vi "Feedback Node - Building an Array.vi"() -> ()   [LabVIEW 2023]
doc: "This VI uses a While Loop with a Feedback Node to build an array of random data. A Waveform Graph displays the array of random data as the array is built."
panel:
  out "Random Data (Shift Register)":dbl[](graph)
  out "Random Data (Feedback Node)":dbl[](graph)
  in  "Stop":bool
  # "Overview: Demonstrates the use of a Feedback Node to store data between iterations of a loop.\nInstructions:\nRun the VI. It will display data accumulated across all iterations of a loop. See the block diagram for more information."
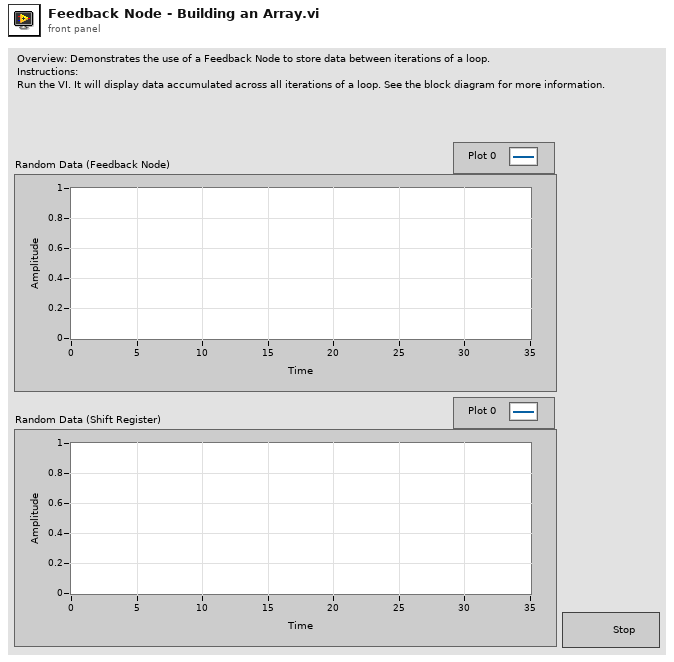
[diagram p1: front panel]
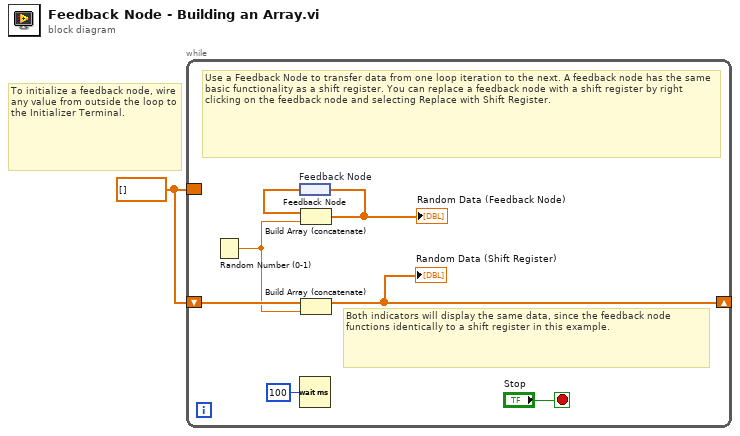
[diagram p0: block diagram]
diagram:
  w1 = dbl[] []
  # "To initialize a feedback node, wire any value from outside the loop to the Initializer Terminal."
  n1 = while {
    border: w1 -> [_]
    shift-right: [w2] -> _
    shift-left: w1 -> [w4]
    stop <- "Stop" stop-if-true
    # "Both indicators will display the same data, since the feedback node functions identically to a shift register in this example."
    # "Use a Feedback Node to transfer data from one loop iteration to the next. A feedback node has the same basic functionality as a shift register. You can replace a feedback node with a shift register by right clicking on the feedback node and selecting Replace with Shift Register."
    n2 = Random Number (0-1)() -> (number: 0 to 1=w3:dbl)
    n3 = feedback #1 "Feedback Node"() -> (w7:dbl[])
    n4 = Wait (ms)(milliseconds to wait=u32 100) -> ()  [unwired: 1 out]
    n5 = Build Array (concatenate)(w7, w3) -> (w6:dbl[])
    "Random Data (Feedback Node)" <- w6
    n6 = feedback-in #1(w6) -> ()
    n7 = Build Array (concatenate)(w4, w3) -> (w2:dbl[])
    "Random Data (Shift Register)" <- w2
  }
